vi "IRSensorConv.vi"(11 "Infrared Sensor Reading":fxp<+/-,25,5>) -> (3 "Sensor Data":dbl)   [LabVIEW 2018, in "kevLib2010.lvlib"]
uses:
  kevLib2010.lvlib
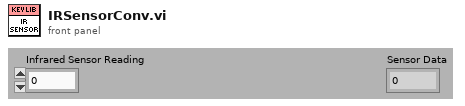
[diagram p1: front panel]
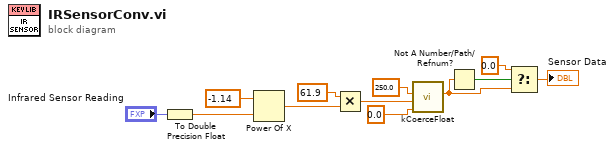
[diagram p0: block diagram]
diagram:
  n1 = To Double Precision Float(number="Infrared Sensor Reading") -> (double precision float=w11:dbl)
  n2 = Power Of X(1:w11, 2:-1.14 ("y")) -> (0:w9:dbl)
  n3 = Multiply(x=61.9, y=w9) -> (x*y=w7:dbl)
  n4 = call "kCoerceFloat.vi"("lower"=0.0, "input"=w7, "upper"=250.0) -> ("output"=w2:dbl)  [unwired: 7 in, 1 out]
  n5 = Not A Number/Path/Refnum?(number/path/refnum=w2) -> (NaN/Path/Refnum?=w4:bool)
  n6 = Select(t=0.0, s=w4, f=w2) -> (s? t:f=→"Sensor Data":dbl)
